vi "FP behavior FWD obstacle avoidance.vi"(1 "Behavior\nVelocity":dbl=20.0, 2 "Activate?":bool=TRUE, 3 "IR Sensors":T1(array[cluster])) -> (0 "Obs Avoid Array":dbl[](array[numeric]))   [LabVIEW 2014]
doc: "This vi uses the values from the Bow sensor to create an Obstacle Avoidance Array."
panel:
  out "Before Scaling":cluster{dbl, dbl, dbl[]}(graph)
  out "Waveform Graph":cluster{dbl, dbl, dbl[]}(graph)
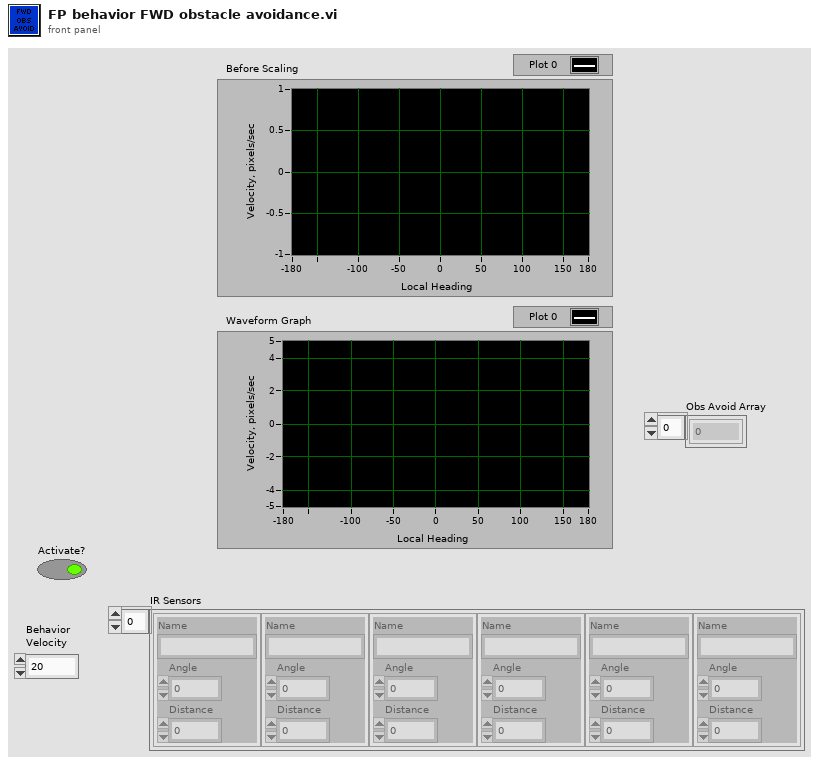
[diagram p1: front panel]
types:
  T1 = cluster{"Name":string, "Angle":dbl, "Distance":dbl}[]
  T2 = cluster{"Name":string, "Angle":dbl, "Distance":dbl}
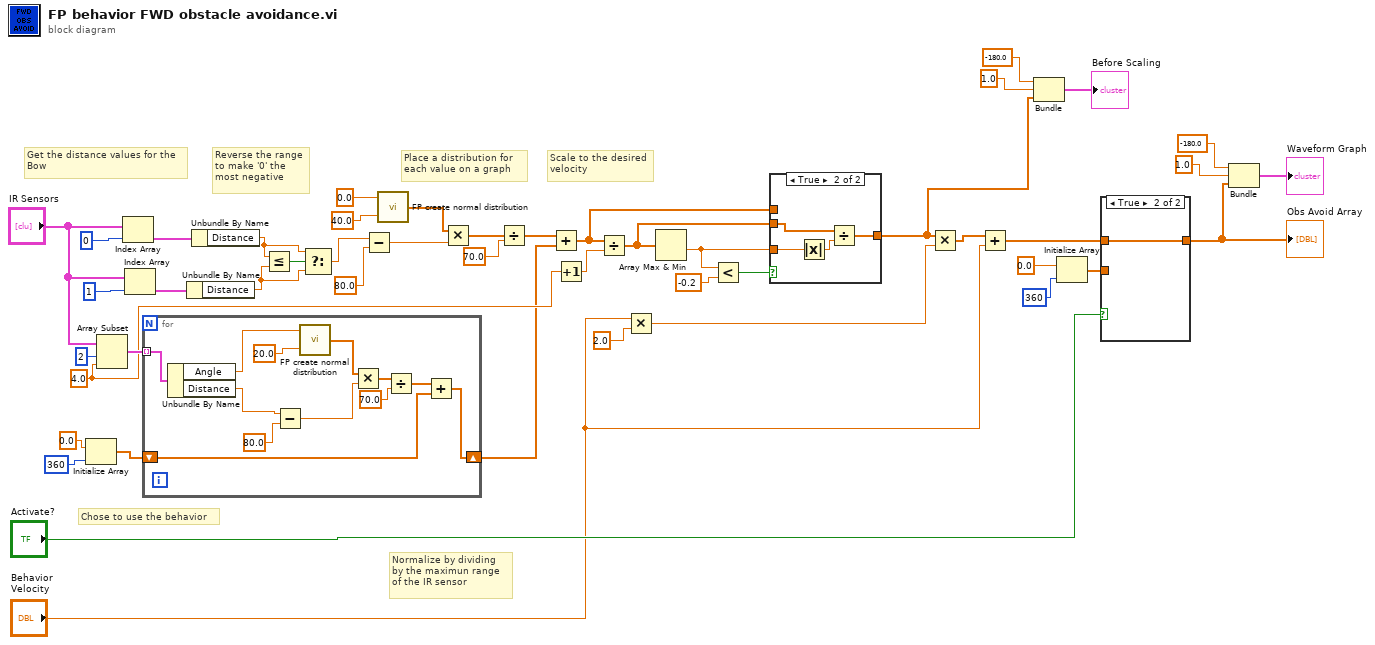
[diagram p0: block diagram]
diagram:
  w19 = 4.0 ("length")
  # "Scale to the desired\nvelocity"
  # "Chose to use the behavior"
  # "Reverse the range\nto make '0' the\nmost negative"
  # "Normalize by dividing\nby the maximun range\nof the IR sensor"
  # "Place a distribution for \neach value on a graph"
  # "Get the distance values for the\nBow"
  n1 = Initialize Array(0.0 ("element"), 360 ("dimension size")) -> (w20:dbl[])
  n2 = Array Subset(array="IR Sensors", index=2, length=w19) -> (w24:T1)
  n3 = Index Array(array="IR Sensors", index=0) -> (element=w46:T2)
  n4 = Index Array(array="IR Sensors", index=1) -> (element=w29:T2)
  n5 = for {
    tunnel: w24 -> [w59] mode=indexing
    shift-right: [w50] -> w9
    shift-left: w20 -> [w51]
    n6 = Unbundle By Name(w59) -> ("Angle"=w57:dbl, "Distance"=w49:dbl)
    n7 = Subtract(x=w49, y=80.0) -> (x-y=w56:dbl)
    n8 = call "FP create normal distribution.vi"("std (Normal)"=20.0, "mean"=w57) -> ("ACT array"=w55:dbl[])
    n9 = Multiply(x=w55, y=w56) -> (x*y=w54:dbl[])
    n10 = Divide(x=w54, y=70.0) -> (x/y=w52:dbl[])
    n11 = Add(x=w52, y=w51) -> (x+y=w50:dbl[])
  }
  n12 = Unbundle By Name(w29) -> ("Distance"=w17:dbl)
  n13 = Unbundle By Name(w46) -> ("Distance"=w27:dbl)
  n14 = Less Or Equal?(x=w27, y=w17) -> (x <= y?=w28:bool)
  n15 = Select(t=w27, s=w28, f=w17) -> (s? t:f=w11:dbl)
  n16 = Subtract(x=w11, y=80.0) -> (x-y=w40:dbl)
  n17 = call "FP create normal distribution.vi"("std (Normal)"=40.0, "mean"=0.0) -> ("ACT array"=w21:dbl[])
  n18 = Multiply(x=w21, y=w40) -> (x*y=w39:dbl[])
  n19 = Divide(x=w39, y=70.0) -> (x/y=w10:dbl[])
  n20 = Add(x=w10, y=w9) -> (x+y=w2:dbl[])
  n21 = Increment(x=w19) -> (x+1=w18:dbl)
  n22 = Divide(x=w2, y=w18) -> (x/y=w1:dbl[])
  n23 = Multiply(x="Behavior\nVelocity", y=2.0) -> (x*y=w32:dbl)
  n24 = Array Max & Min(array=w1) -> (min value=w5:dbl)  [unwired: 3 out]
  n25 = Less?(x=w5, y=-0.2) -> (x < y?=w3:bool)
  n26 = case shown="True" w3 {
    tunnel: w2 -> [w60 _]
    tunnel: [w60 w64] -> w6
    tunnel: w5 -> [_ w62]
    tunnel: w1 -> [_ w61]
    frame False {
    }
    frame True {
      n27 = Absolute Value(x=w62) -> (abs(x)=w63:dbl)
      n28 = Divide(x=w61, y=w63) -> (x/y=w64:dbl[])
    }
  }
  n29 = Multiply(x=w6, y=w32) -> (x*y=w15:dbl[])
  n30 = Add(x=w15, y="Behavior\nVelocity") -> (x+y=w7:dbl[])
  n31 = Bundle(-180.0, 1.0, w6) -> (→"Before Scaling":cluster{dbl, dbl, dbl[]})  [unwired: 1 in]
  n32 = Initialize Array(0.0 ("element"), 360 ("dimension size")) -> (w35:dbl[])
  n33 = case shown="True" "Activate?" {
    tunnel: w7 -> [_ w66]
    tunnel: w35 -> [w65 _]
    tunnel: [w65 w66] -> w34
    frame False {
    }
    frame True {
    }
  }
  "Obs Avoid Array" <- w34
  n34 = Bundle(-180.0, 1.0, w34) -> (→"Waveform Graph":cluster{dbl, dbl, dbl[]})  [unwired: 1 in]
